vi "Prober_InitialiseUI.vi"(8 "error in (no error)":errorcluster, 11 "SemiProbe in":refnum<class "SemiProbe.lvclass">) -> (0 "error out":errorcluster, 2 "Probestation Configuration":variant, 3 "SemiProbe out":refnum<class "SemiProbe.lvclass">)   [LabVIEW 2013, in "SemiProbe.lvclass"]
uses:
  SemiProbe.lvclass
  SemiProbe.vi
  <vilib>/Instr/_visa.llb/VISA Configure Serial Port (Instr).vi
panel:
  in  "port":u16=5050
  in  "address":string="localhost"
  in  "OK Button":bool
  in  "Cancel":bool
  in  "VISA In":refnum<visa-resource-name> caption="address"
  in  "SP Software Running":bool
  in  "Local":bool
  out "Cancelled":bool
  # "SemiProbe Initialization"
  # "Confirm that the SemiProbe applications are running and configured.\n\n1) Run Navigator, SemiServer, Prober Interface, Communications Controller\n2) Configure Communications Controller: \n   a) (com port, stop bits, start bits, parity, baud rate) =                               \n      (COM6, 1, 8, None, 9600)\n   b) Incoming/Outgoing EOL = Lf\n   c) RS232 Checked.\n\nCaution the chuck will move down and to center and z heights will be cleared."
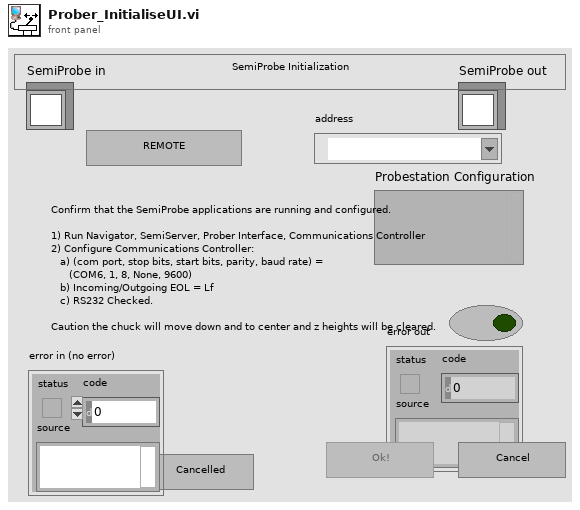
[diagram p1: front panel]
types:
  T1 = cluster{"SP Local":bool, "SP Min Usable Z":dbl, "SP REMOTE Comm Parameters":cluster{"SemiProbe VISA":refnum<visa-resource-name>, "write delay(ms)":i32, "buffer is full loop multiplicity":i32, "read threshold check rate (ms)":u32}, "SP Comm Params":cluster{"LF as Return EOL":bool, "SP Error Debug":bool}, "SP LOCAL Comm Parameters":cluster{"address":string, "port":i32, "SP TCP Cnx ID":refnum<k5>, "mode (standard)":enum16{"Standard", "Buffered", "CRLF", "Immediate"}, "bytes to read":i32, "timeout (ms)":i32}, "SP Operation Parameters":cluster{"SP Load Less Than Thr?":bool, "SP Load Threshold (um)":dbl, "SP Current Location":cluster{"X (um)":ext, "Y (um)":ext, "Z (um)":ext, "T (degree)":ext}, "SP Chuck Speeds":cluster{"XY Speed (10-100%)":dbl, "Z Speed (10-100%)":dbl, "T Speed (10-100%)":dbl}, "Manual Step Parameters":cluster{"Step in X":bool, "X S-Speed [µm/step]":sgl, "Step in Y":bool, "Y S-Speed [µm/step]":sgl, "Step in Z":bool, "Z S-Speed [µm/step]":sgl, "Step in T":bool, "T S-Speed [mdegree/step]":sgl, "X Increase":bool, "Y Increase?":bool, "Z Increase?":bool, "T Increase?":bool}, "Z Stepper":cluster{"UP/DOWN":bool, "UP/DOWN Speed [µm/step]":i32, "SP Z Step":bool}, "Z Heights Set":bool, "SP Contact Search":cluster{"Contact Circuit":enum16{"12", "1", "2"}, "Speed [1000-10000]":sgl, "Start Height [µm]":sgl, "Search Band [µm]":sgl, "Overdrive [µm]":sgl}, "Separation Distance [µm]":u32, "Contact Height [µm]":u32, "Use Overdrive?":bool, "Touchdown method":enum16{"no feedback", "Arduino edgesense", "SP contact circuit"}, "Arduino Edgesense params":cluster{"touchdown height [µm]":i32, "search band [µm]":u32, "speed [µm/step]":u32, "overdrive [µm]":u32}}}
  T2 = cluster{"SemiProbe VISA":refnum<visa-resource-name>, "write delay(ms)":i32, "buffer is full loop multiplicity":i32, "read threshold check rate (ms)":u32}
  T3 = cluster{"address":string, "port":i32, "SP TCP Cnx ID":refnum<k5>, "mode (standard)":enum16{"Standard", "Buffered", "CRLF", "Immediate"}, "bytes to read":i32, "timeout (ms)":i32}
  T4 = cluster{"SP Load Less Than Thr?":bool, "SP Load Threshold (um)":dbl, "SP Current Location":cluster{"X (um)":ext, "Y (um)":ext, "Z (um)":ext, "T (degree)":ext}, "SP Chuck Speeds":cluster{"XY Speed (10-100%)":dbl, "Z Speed (10-100%)":dbl, "T Speed (10-100%)":dbl}, "Manual Step Parameters":cluster{"Step in X":bool, "X S-Speed [µm/step]":sgl, "Step in Y":bool, "Y S-Speed [µm/step]":sgl, "Step in Z":bool, "Z S-Speed [µm/step]":sgl, "Step in T":bool, "T S-Speed [mdegree/step]":sgl, "X Increase":bool, "Y Increase?":bool, "Z Increase?":bool, "T Increase?":bool}, "Z Stepper":cluster{"UP/DOWN":bool, "UP/DOWN Speed [µm/step]":i32, "SP Z Step":bool}, "Z Heights Set":bool, "SP Contact Search":cluster{"Contact Circuit":enum16{"12", "1", "2"}, "Speed [1000-10000]":sgl, "Start Height [µm]":sgl, "Search Band [µm]":sgl, "Overdrive [µm]":sgl}, "Separation Distance [µm]":u32, "Contact Height [µm]":u32, "Use Overdrive?":bool, "Touchdown method":enum16{"no feedback", "Arduino edgesense", "SP contact circuit"}, "Arduino Edgesense params":cluster{"touchdown height [µm]":i32, "search band [µm]":u32, "speed [µm/step]":u32, "overdrive [µm]":u32}}
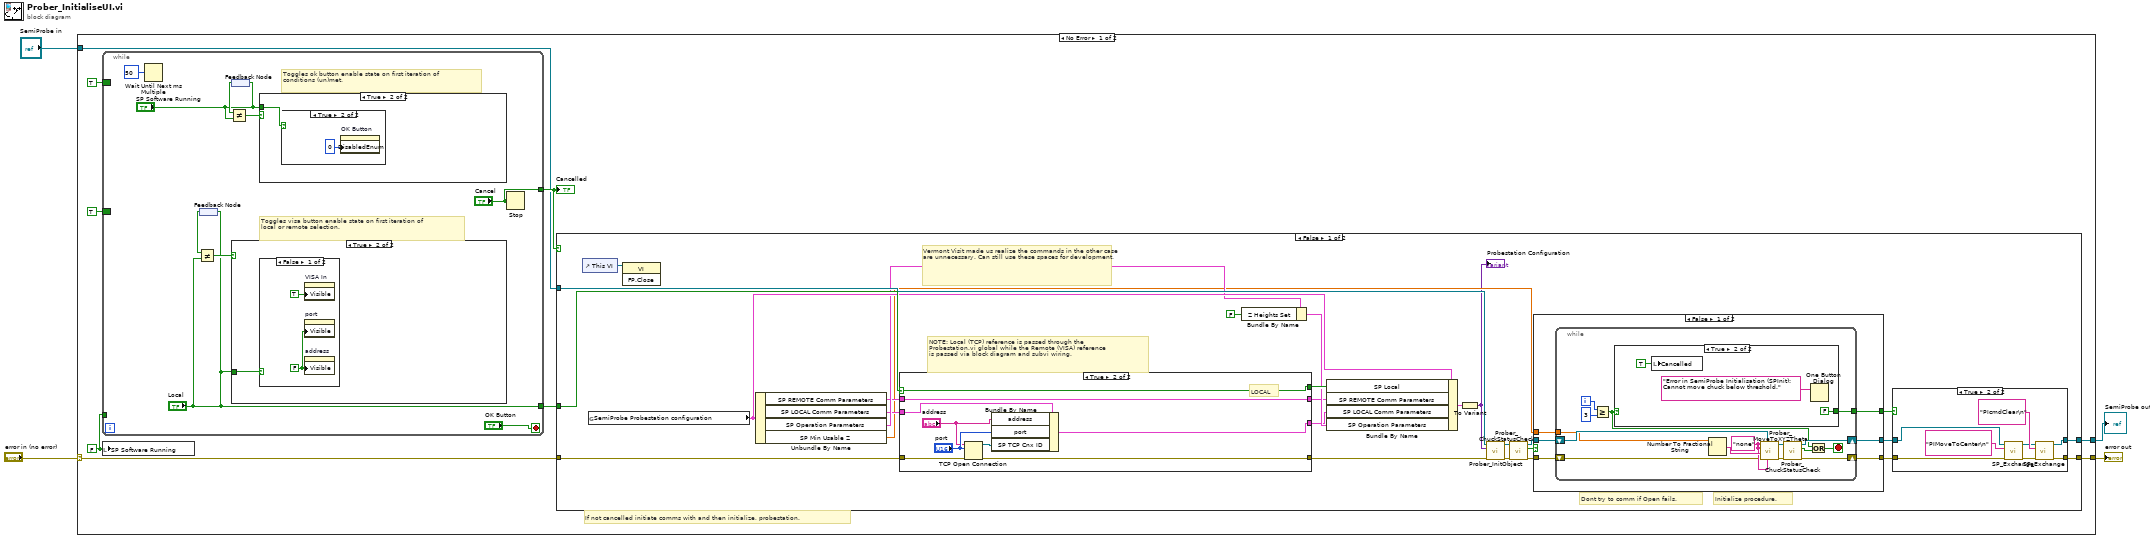
[diagram p0: block diagram]
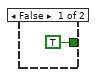
[diagram p2: hidden frame]
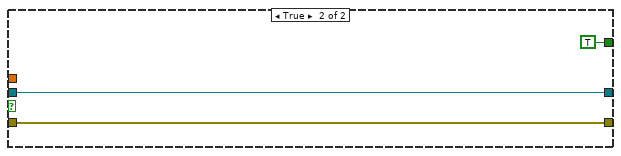
[diagram p3: hidden frame]
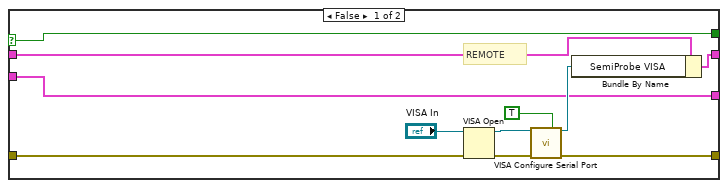
[diagram p5: hidden frame]
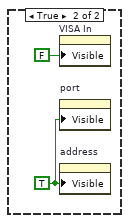
[diagram p8: hidden frame]
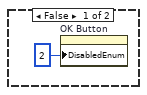
[diagram p10: hidden frame]
diagram:
  n1 = case shown="No Error" "error in (no error)" {
    selector: "error in (no error)" -> [w7 w119]
    tunnel: [w8 w119] -> w3
    tunnel: "SemiProbe in" -> [w6 w118]
    tunnel: [w5 w118] -> w1
    frame No Error {
      w10 = FALSE
      # "If not cancelled initiate comms with and then initialize, probestation."
      n2 = while {
        tunnel: ["Cancel"] -> w12
        border: TRUE -> [_]
        tunnel: w10 -> [_]
        border: TRUE -> [_]
        tunnel: ["Local"] -> w13
        stop <- "OK Button" stop-if-true
        # "Toggles visa button enable state on first iteration of \nlocal or remote selection."
        # "Toggles ok button enable state on first iteration of \nconditions (un)met."
        n3 = Wait Until Next ms Multiple(millisecond multiple=u32 50) -> ()  [unwired: 1 out]
        n4 = feedback #1() -> (w104:bool)
        n5 = Not Equal?(x=w104, y="Local") -> (x != y?=w105:bool)
        n6 = feedback-in #1("Local") -> ()
        n7 = feedback-in #2("SP Software Running") -> ()
        n8 = feedback #2() -> (w108:bool)
        n9 = Not Equal?(x=w108, y="SP Software Running") -> (x != y?=w107:bool)
        n10 = case shown="True" w105 {
          tunnel: "Local" -> [_ w110]
          frame False {
          }
          frame True {
            n11 = case shown="False" w110 {
              frame False {
                w112 = FALSE
                n12 = property on="VISA In" class="VISAName"("Visible"=TRUE) -> ()  [unwired: 2 in, 2 out]
                n13 = property on="port" class="DigNum (strict)"("Visible"=w112) -> ()  [unwired: 2 in, 2 out]
                n14 = property on="address" class="Str"("Visible"=w112) -> ()  [unwired: 2 in, 2 out]
              }
              frame True {
                w114 = TRUE
                n15 = property on="VISA In" class="VISAName"("Visible"=FALSE) -> ()  [unwired: 2 in, 2 out]
                n16 = property on="port" class="DigNum (strict)"("Visible"=w114) -> ()  [unwired: 2 in, 2 out]
                n17 = property on="address" class="Str"("Visible"=w114) -> ()  [unwired: 2 in, 2 out]
              }
            }
          }
        }
        n18 = case shown="True" w107 {
          tunnel: "SP Software Running" -> [_ w115]
          frame False {
          }
          frame True {
            n19 = case shown="True" w115 {
              frame False {
                n20 = property on="OK Button" class="Bool"("DisabledEnum"=2) -> ()  [unwired: 2 in, 2 out]
              }
              frame True {
                n21 = property on="OK Button" class="Bool"("DisabledEnum"=0) -> ()  [unwired: 2 in, 2 out]
              }
            }
          }
        }
        n22 = Stop(stop? (T)="Cancel") -> ()
      }
      "Cancelled" <- w12
      n23 = local write "SP Software Running"(w10) -> ()
      n24 = case shown="False" w12 {
        tunnel: [w40 w99] -> w5
        tunnel: w13 -> [w38 _]
        tunnel: [w37 w100] -> w8
        tunnel: w7 -> [w36 w100]
        tunnel: w6 -> [w25 w99]
        frame False {
          # "Vermont Visit made us realize the commands in the other case are unnecessary. Can still use these spaces for development."
          # "Initialize procedure."
          # "NOTE: Local (TCP) reference is passed through the \nProbestation.vi global while the Remote (VISA) reference\nis passed via block diagram and subvi wiring."
          # "Dont try to comm if Open fails."
          n25 = control-ref of="This VI"() -> (w39:refnum<vi>)
          n26 = global read "SemiProbe.vi" "SemiProbe Probestation configuration"() -> (w22:T1)
          n27 = invoke class="VI" method="FP.Close"(reference=w39) -> ()  [unwired: 2 in, 3 out]
          n28 = Unbundle By Name(w22) -> ("SP REMOTE Comm Parameters"=w19:T2, "SP LOCAL Comm Parameters"=w18:T3, "SP Operation Parameters"=w21:T4, "SP Min Usable Z"=w15:dbl)
          n29 = case shown="True" w38 {
            selector: w38 -> [w84 w92]
            tunnel: [w88 w97] -> w24
            tunnel: w36 -> [w85 w98]
            tunnel: [w84 w92] -> w29
            tunnel: [w79 w93] -> w16
            tunnel: [w82 w90] -> w17
            tunnel: w19 -> [w80 w90]
            tunnel: w18 -> [w79 w91]
            frame False {
              # "REMOTE"
              n30 = VISA Open(error in (no error)=w85, VISA resource name="VISA In") -> (VISA resource name=w83:refnum<visa-resource-name>, error out=w89:errorcluster)  [unwired: 3 in]
              n31 = call-poly "VISA Configure Serial Port"("VISA resource name"=w83, "Enable Termination\nChar (T)"=TRUE, "error in (no error)"=w89) -> ("VISA resource name out"=w81:refnum<visa-resource-name>, "error out"=w88:errorcluster)  [unwired: 11 in]
              n32 = Bundle By Name(cluster=w80, "SemiProbe VISA"=w81) -> (w82:T2)
            }
            frame True {
              # "LOCAL"
              n33 = TCP Open Connection(address="address", remote port or service name="port", error in (no error)=w98) -> (connection ID=w96:refnum<k5>, error out=w97:errorcluster)  [unwired: 2 out]
              n34 = Bundle By Name(cluster=w91, "address"="address", "port"="port", "SP TCP Cnx ID"=w96) -> (w93:T3)
            }
          }
          n35 = Bundle By Name(cluster=w21, "Z Heights Set"=FALSE) -> (w20:T4)
          n36 = Bundle By Name(cluster=w22, "SP Local"=w29, "SP REMOTE Comm Parameters"=w17, "SP LOCAL Comm Parameters"=w16, "SP Operation Parameters"=w20) -> (w28:T1)
          n37 = To Variant(anything=w28) -> (Variant=w14:variant)
          "Probestation Configuration" <- w14
          n38 = call-dynamic "Prober_InitObject.vi"("error in (no error)"=w24, "Prober Configuration"=w14, "SemiProbe in"=w25) -> ("error out"=w27:errorcluster, "SemiProbe out"=w26:refnum<class "SemiProbe.lvclass">)  [unwired: 7 in]
          n39 = call-dynamic "Prober_ChuckStatusCheck.vi"("error in (no error)"=w27, "SemiProbe in"=w26) -> ("error out"=w32:errorcluster, "Chuck at CONTACT?"=w30:bool, "SemiProbe out"=w31:refnum<class "SemiProbe.lvclass">)  [unwired: 7 in]
          n40 = case shown="False" w30 {
            tunnel: [w46 w68] -> w35
            tunnel: [w45 w67] -> w34
            tunnel: [w44 TRUE] -> w33
            tunnel: w32 -> [w43 w68]
            tunnel: w31 -> [w42 w67]
            tunnel: w15 -> [w41 _]
            frame False {
              n41 = while {
                shift-right: [w55] -> w46
                shift-left: w43 -> [w59]
                shift-right: [w54] -> w45
                shift-left: w42 -> [w58]
                tunnel: [w50] -> w44
                tunnel: w41 -> [w47]
                i -> [w52]
                stop <- w49 stop-if-true
                w60 = "none" ("Error String IN")
                n42 = Greater Or Equal?(x=w52, y=3) -> (x >= y?=w48:bool)
                n43 = case shown="True" w48 {
                  tunnel: [TRUE FALSE] -> w50
                  frame False {
                  }
                  frame True {
                    n44 = local write "Cancelled"(TRUE) -> ()
                    n45 = One Button Dialog(message="Error in SemiProbe Initialisation (SPInit): Cannot move chuck below threshold.") -> ()  [unwired: 1 in, 1 out]
                  }
                }
                n46 = Number To Fractional String(number=w47) -> (F-format string=w61:string)  [unwired: 3 in]
                n47 = call-dynamic "Prober_MoveToXYZTheta.vi"("Theta location [mdeg]"=w60, "SemiProbe in"=w58, "error in (no error)"=w59, "Z location [µm]"=w61, "Y location [µm]"=w60, "X location [µm]"=w60) -> ("error out"=w57:errorcluster, "SemiProbe out"=w56:refnum<class "SemiProbe.lvclass">)  [unwired: 3 in, 1 out]
                n48 = call-dynamic "Prober_ChuckStatusCheck.vi"("error in (no error)"=w57, "SemiProbe in"=w56) -> ("error out"=w55:errorcluster, "Chuck at CONTACT?"=w53:bool, "SemiProbe out"=w54:refnum<class "SemiProbe.lvclass">)  [unwired: 7 in]
                n49 = Or(x=w48, y=w53) -> (x .or. y?=w49:bool)
              }
            }
            frame True {
            }
          }
          n50 = case shown="True" w33 {
            tunnel: [w70 w74] -> w37
            tunnel: [w69 w73] -> w40
            tunnel: w35 -> [w70 w72]
            tunnel: w34 -> [w69 w71]
            frame False {
              # "Cancellled due to z lowering error."
            }
            frame True {
              n51 = call-dynamic "SP_Exchange.vi"("error in (no error)"=w72, "command"="PIMoveToCenter\n" ("Error String IN"), "SemiProbe in"=w71) -> ("error out"=w76:errorcluster, "SemiProbe out"=w75:refnum<class "SemiProbe.lvclass">)  [unwired: 4 in, 3 out]
              n52 = call-dynamic "SP_Exchange.vi"("error in (no error)"=w76, "command"="PIcmdClear\n" ("Error String IN"), "SemiProbe in"=w75) -> ("error out"=w74:errorcluster, "SemiProbe out"=w73:refnum<class "SemiProbe.lvclass">)  [unwired: 4 in, 3 out]
            }
          }
        }
        frame True {
        }
      }
    }
    frame Error {
    }
  }
  "error out" <- w3
  "SemiProbe out" <- w1
